vi "Write Phase Value.vi"(10 "Phase Value":cluster{"Phase Value":dbl, "Random":bool}, 11 "MCCW ACLR in":refnum<class "MCCW ACLR.lvclass">) -> (3 "MCCW ACLR out":refnum<class "MCCW ACLR.lvclass">)   [LabVIEW 2020, in "MCCW ACLR.lvclass"]
uses:
  MCCW ACLR.lvclass
  MCCW ACLR.lvclass/MCCW ACLR.ctl
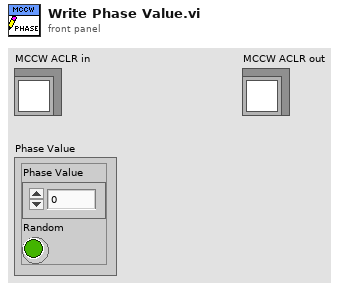
[diagram p1: front panel]
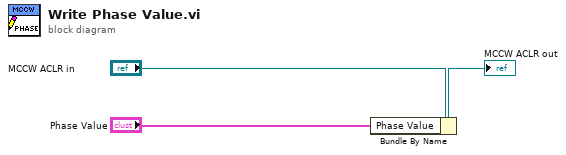
[diagram p0: block diagram]
diagram:
  n1 = Bundle By Name(cluster="MCCW ACLR in", "Phase Value"="Phase Value") -> (→"MCCW ACLR out":refnum<class "MCCW ACLR.lvclass">)
